vi "WaypointGoodnessAtHeading.vi"(10 "Waypoint Direction":i32, 11 "Heading":i32) -> (3 "Waypoint goodness\nat this heading":sgl)   [LabVIEW 2011]
panel:
  out "Angle in radians":sgl
  out "cos(x)":sgl
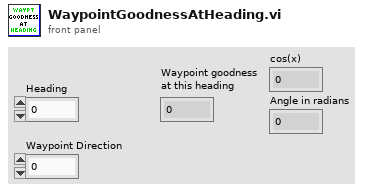
[diagram p1: front panel]
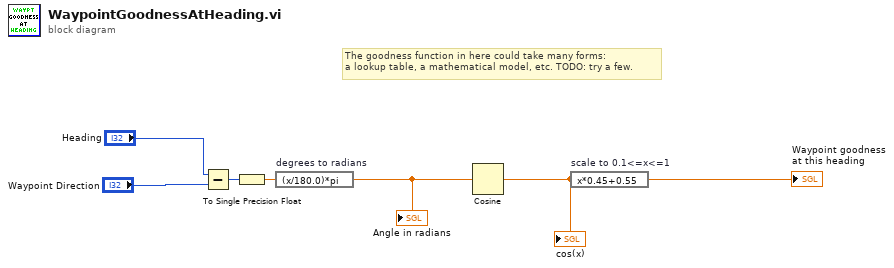
[diagram p0: block diagram]
diagram:
  # "The goodness function in here could take many forms:\na lookup table, a mathematical model, etc. TODO: try a few."
  n1 = Subtract(x="Heading", y="Waypoint Direction") -> (x-y=w3:i32)
  n2 = To Single Precision Float(number=w3) -> (single precision float=w5:sgl)
  n3 = expression code="(x/180.0)*pi" "degrees to radians"(w5) -> (w4:sgl)
  "Angle in radians" <- w4
  n4 = Cosine(x=w4) -> (cos(x)=w2:sgl)
  "cos(x)" <- w2
  n5 = expression code="x*0.45+0.55" "scale to 0.1<=x<=1"(w2) -> (→"Waypoint goodness\nat this heading":sgl)
